vi "RecipeIndexControl.vi"(6 "Index_List":i32[](array[numeric]), 8 "error in (no error)":errorcluster, 10 "Recipe_Input":string[][](array[string])) -> (0 "error out":errorcluster, 1 "Status":string, 4 "Index_List_out":i32[](array[numeric]))   [LabVIEW 2014]
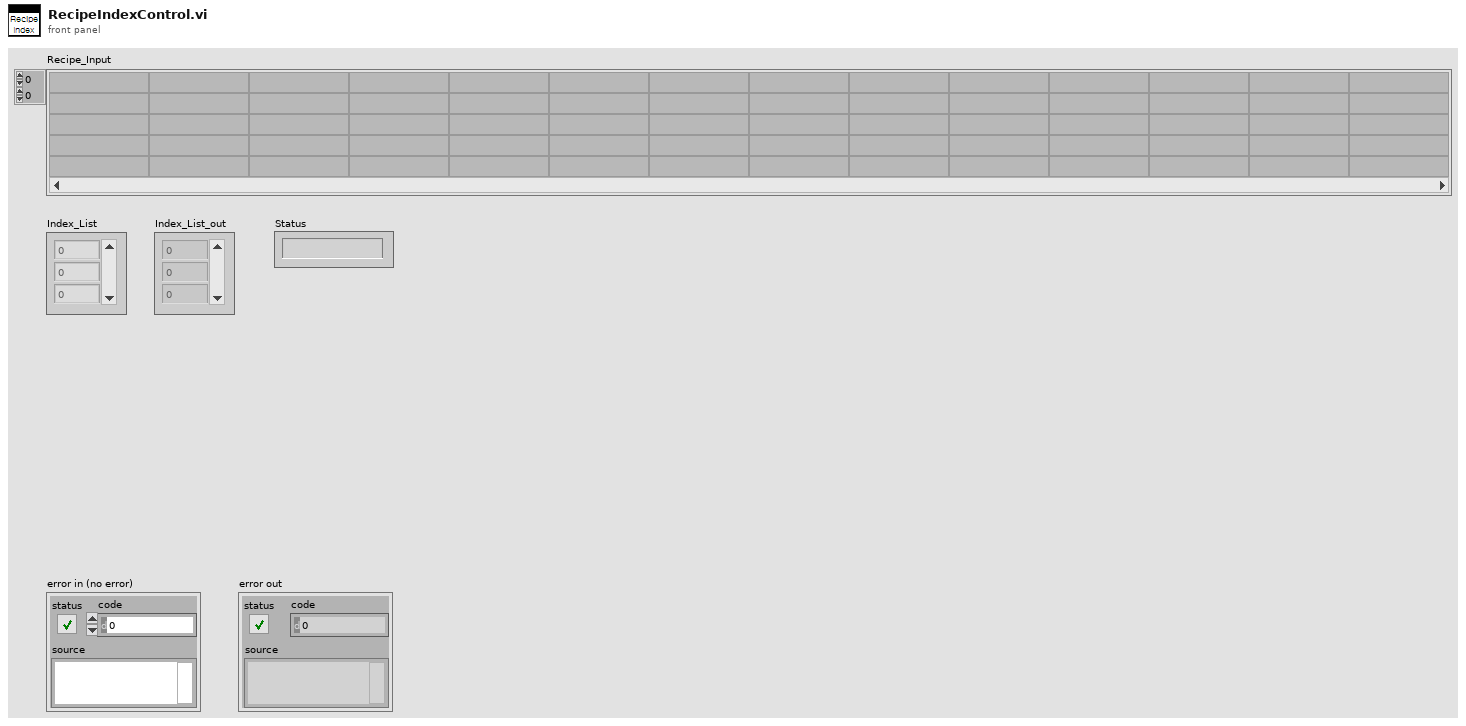
[diagram p1: front panel]
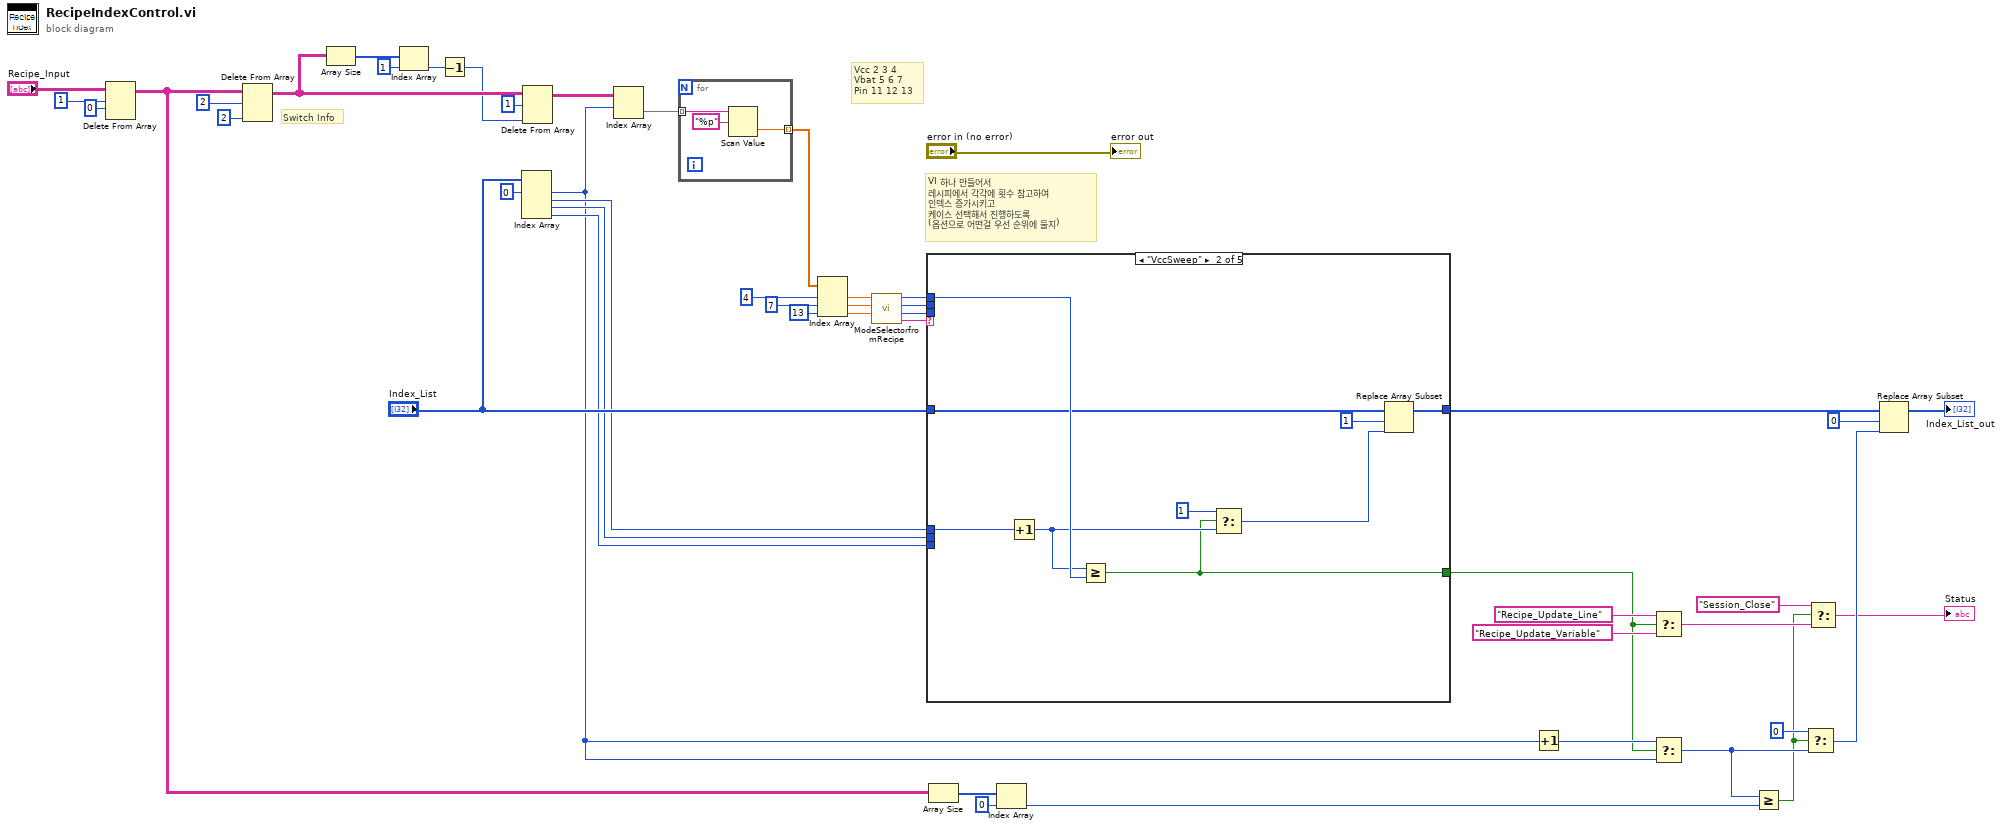
[diagram p0: block diagram]
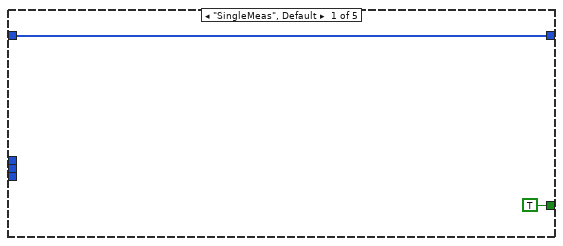
[diagram p2: hidden frame]
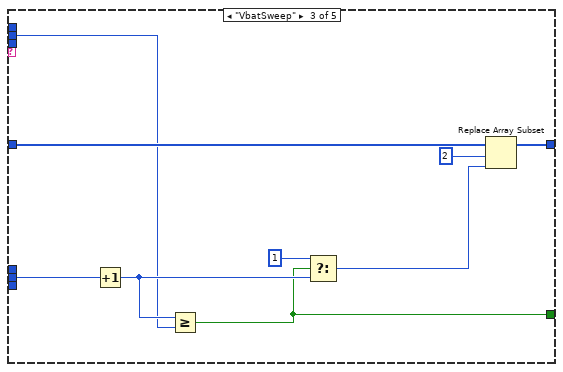
[diagram p3: hidden frame]
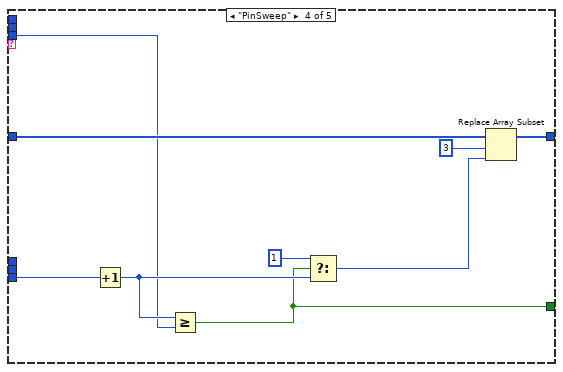
[diagram p4: hidden frame]
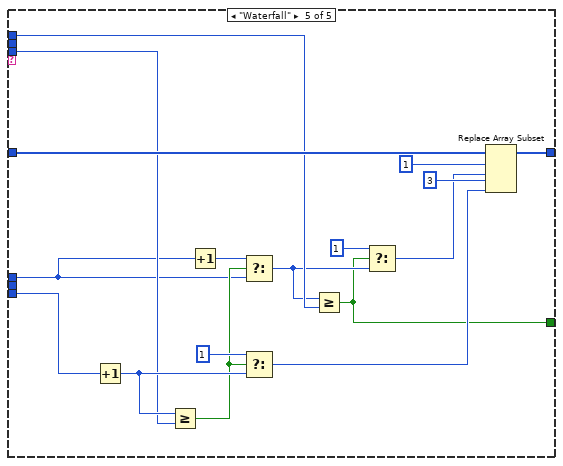
[diagram p5: hidden frame]
diagram:
  # "VI 하나 만들어서 \n레시피에서 각각에 횟수 참고하여\n인덱스 증가시키고\n케이스 선택해서 진행하도록\n(옵션으로 어떤걸 우선 순위에 둘지)"
  # "Vcc 2 3 4\nVbat 5 6 7\nPin 11 12 13"
  # "Switch Info"
  n1 = Delete From Array(array="Recipe_Input", length=1, index (row)=0) -> (array with subset deleted=w12:string[][])  [unwired: 1 in, 1 out]
  n2 = Delete From Array(array=w12, length=2, index (col)=2 ("disabled index (col)")) -> (array with subset deleted=w42:string[][])  [unwired: 1 in, 1 out]
  n3 = Array Size(array=w42) -> (size(s)=w44:i32[])
  n4 = Index Array(array=w44, index=1) -> (element=w41:i32)
  n5 = Decrement(x=w41) -> (x-1=w39:i32)
  n6 = Index Array(array="Index_List", index #1=0 ("index")) -> (element #1=w15:i32, element #2=w20:i32, element #3=w19:i32, element #4=w18:i32)  [unwired: 3 in]
  n7 = Delete From Array(array=w42, length=1, index (col)=w39) -> (array with subset deleted=w38:string[][])  [unwired: 1 in, 1 out]
  n8 = Index Array(array=w38, index (row)=w15) -> (element=w37:string[])  [unwired: 1 in]
  n9 = for {
    tunnel: w37 -> [w52] mode=indexing
    tunnel: [w50] -> w34 mode=indexing
    n10 = Scan Value(string=w52, format string="%p") -> (value=w50:dbl)  [unwired: 1 in, 1 out]
  }
  n11 = Index Array(array=w34, index #1=4 ("index"), index #2=7 ("index"), index #3=13 ("index")) -> (element #1=w30:dbl, element #2=w29:dbl, element #3=w28:dbl)
  n12 = call "ModeSelectorfromRecipe.vi"("Pin_Index"=w28, "Vbat_Index"=w29, "Vcc_Index"=w30) -> ("Mode"=w24:string, "Pin_Index 2"=w25:i32, "Vbat_Index 2"=w26:i32, "Vcc_Index 2"=w27:i32)  [unwired: 5 in]
  n13 = case shown="\"VccSweep\"" w24 {
    tunnel: w27 -> [_ w62 _ _ w86]
    tunnel: w26 -> [_ _ w65 _ _]
    tunnel: w25 -> [_ _ _ w74 w92]
    tunnel: w18 -> [_ _ _ w75 w93]
    tunnel: w19 -> [_ _ w66 _ _]
    tunnel: w20 -> [_ w63 _ _ w88]
    tunnel: "Index_List" -> [w54 w60 w71 w80 w97]
    tunnel: [w54 w56 w67 w76 w94] -> w17
    tunnel: [TRUE w55 w64 w73 w82] -> w13
    frame "SingleMeas", Default {
    }
    frame "VccSweep" {
      n14 = Increment(x=w63) -> (x+1=w59:i32)
      n15 = Greater Or Equal?(x=w59, y=w62) -> (x >= y?=w55:bool)
      n16 = Select(t=1, s=w55, f=w59) -> (s? t:f=w57:i32)
      n17 = Replace Array Subset(array=w60, new element=w57, index=1) -> (w56:i32[])
    }
    frame "VbatSweep" {
      n18 = Increment(x=w66) -> (x+1=w70:i32)
      n19 = Greater Or Equal?(x=w70, y=w65) -> (x >= y?=w64:bool)
      n20 = Select(t=1, s=w64, f=w70) -> (s? t:f=w68:i32)
      n21 = Replace Array Subset(array=w71, new element=w68, index=2) -> (w67:i32[])
    }
    frame "PinSweep" {
      n22 = Increment(x=w75) -> (x+1=w79:i32)
      n23 = Greater Or Equal?(x=w79, y=w74) -> (x >= y?=w73:bool)
      n24 = Select(t=1, s=w73, f=w79) -> (s? t:f=w77:i32)
      n25 = Replace Array Subset(array=w80, new element=w77, index=3) -> (w76:i32[])
    }
    frame "Waterfall" {
      n26 = Increment(x=w93) -> (x+1=w96:i32)
      n27 = Greater Or Equal?(x=w96, y=w92) -> (x >= y?=w89:bool)
      n28 = Increment(x=w88) -> (x+1=w87:i32)
      n29 = Select(t=w87, s=w89, f=w88) -> (s? t:f=w85:i32)
      n30 = Select(t=1, s=w89, f=w96) -> (s? t:f=w90:i32)
      n31 = Greater Or Equal?(x=w85, y=w86) -> (x >= y?=w82:bool)
      n32 = Select(t=1, s=w82, f=w85) -> (s? t:f=w83:i32)
      n33 = Replace Array Subset(array=w97, new element #1=w83, index #1=1 ("index"), new element #2=w90, index #2=3 ("index")) -> (w94:i32[])
    }
  }
  n34 = Array Size(array=w12) -> (size(s)=w11:i32[])
  n35 = Index Array(array=w11, index=0) -> (element=w9:i32)
  n36 = Increment(x=w15) -> (x+1=w14:i32)
  n37 = Select(t="Recipe_Update_Line", s=w13, f="Recipe_Update_Variable") -> (s? t:f=w5:string)
  n38 = Select(t=w14, s=w13, f=w15) -> (s? t:f=w8:i32)
  n39 = Greater Or Equal?(x=w8, y=w9) -> (x >= y?=w4:bool)
  n40 = Select(t=0, s=w4, f=w8) -> (s? t:f=w6:i32)
  n41 = Select(t="Session_Close", s=w4, f=w5) -> (s? t:f=→"Status":string)
  n42 = Replace Array Subset(array=w17, new element=w6, index=0) -> (→"Index_List_out":i32[])
  "error out" <- "error in (no error)"
